vi "SP Read Single.vi"(8 "error in":errorcluster, 9 "Channel Index":i32=1, 11 "Voltage Setpoint in":refnum<class "Voltage Setpoint.lvclass">) -> (0 "error out":errorcluster, 1 "Changed or First Call?":bool, 2 "Voltage SP":dbl, 3 "Voltage Setpoint out":refnum<class "Voltage Setpoint.lvclass">)   [LabVIEW 2023, in "Voltage Setpoint.lvclass"]
uses:
  Voltage Setpoint.lvclass
  Parents/Setpoint/Setpoint.lvclass
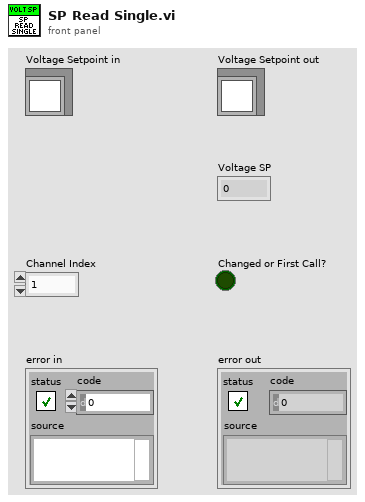
[diagram p1: front panel]
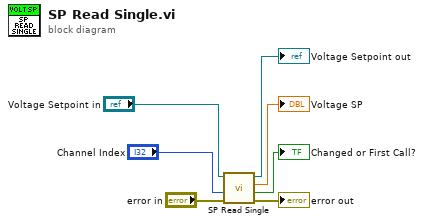
[diagram p0: block diagram]
diagram:
  n1 = call-parent "SP Read Single.vi"("error in"="error in", "Channel Index"="Channel Index", "Setpoint in"="Voltage Setpoint in") -> ("error out"=→"error out":errorcluster, "Changed or First Call?"=→"Changed or First Call?":bool, "Current SP"=→"Voltage SP":dbl, "Setpoint out"=→"Voltage Setpoint out":refnum<class "Voltage Setpoint.lvclass">)  [unwired: 5 in]
